vi "数据主动和反控发送.vi"() -> ()   [LabVIEW 2016, in "数据传输系统.lvlib"]
uses:
  <vilib>/ptbypt/NI_PtbyPt.lvlib
panel:
  out "QN":string
  out "队列中元素数量":i32
  out "元素":cluster{"命令编码CN":string, "QN":string}[](array[cluster])
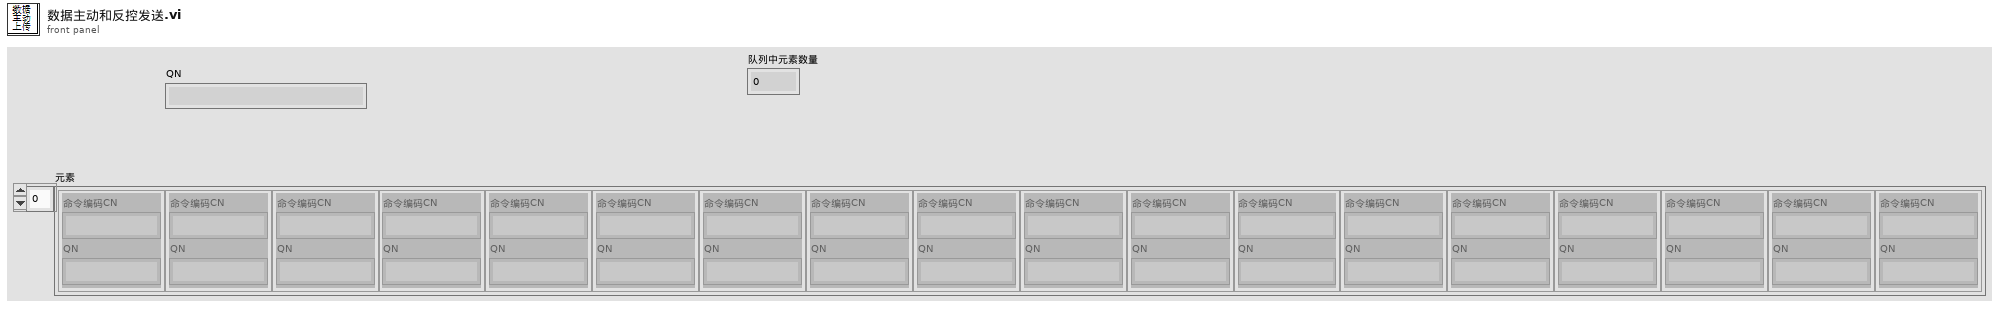
[diagram p1: front panel]
types:
  T1 = cluster{"setini":string, "sysini":string, "hechaini":string, "actualwrite":string, "actualread":string, "datasent":string, "反控命令信息队列":string, "反控与仪器交互":string}
  T2 = enum16{"00点", "01点", "02点", "03点", "04点", "05点", "06点", "07点", "08点", "09点", "10点", "11点", "12点", "13点", "14点", "15点", "16点", "17点", "18点", "19点", "20点", "21点", "22点", "23点"}
  T3 = enum16{"关闭", "星期日", "星期一", "星期二", "星期三", "星期四", "星期五", "星期六"}
  T4 = typedef "LVDateTimeRec.ctl" = cluster{"秒数的小数部分":dbl, "秒":i32, "分":i32, "时":i32, "日":i32, "月":i32, "年":i32, "天数（周）":i32, "天数（年）":i32, "DST":i32}
  T5 = cluster{"[0]":string, "[1]":string, "[2]":string, "[3]":string, "[4]":string, "[5]":string, "[6]":string, "[7]":string, "[8]":string, "[9]":string, "[10]":string, "[11]":string, "[12]":string, "[13]":string, "[14]":string, "[15]":string, "[16]":string, "[17]":string, "[18]":string, "[19]":string, "[20]":string, "[21]":string, "[22]":string, "[23]":string, "[24]":string, "[25]":string, "[26]":string, "[27]":string, "[28]":string, "[29]":string, "[30]":string}
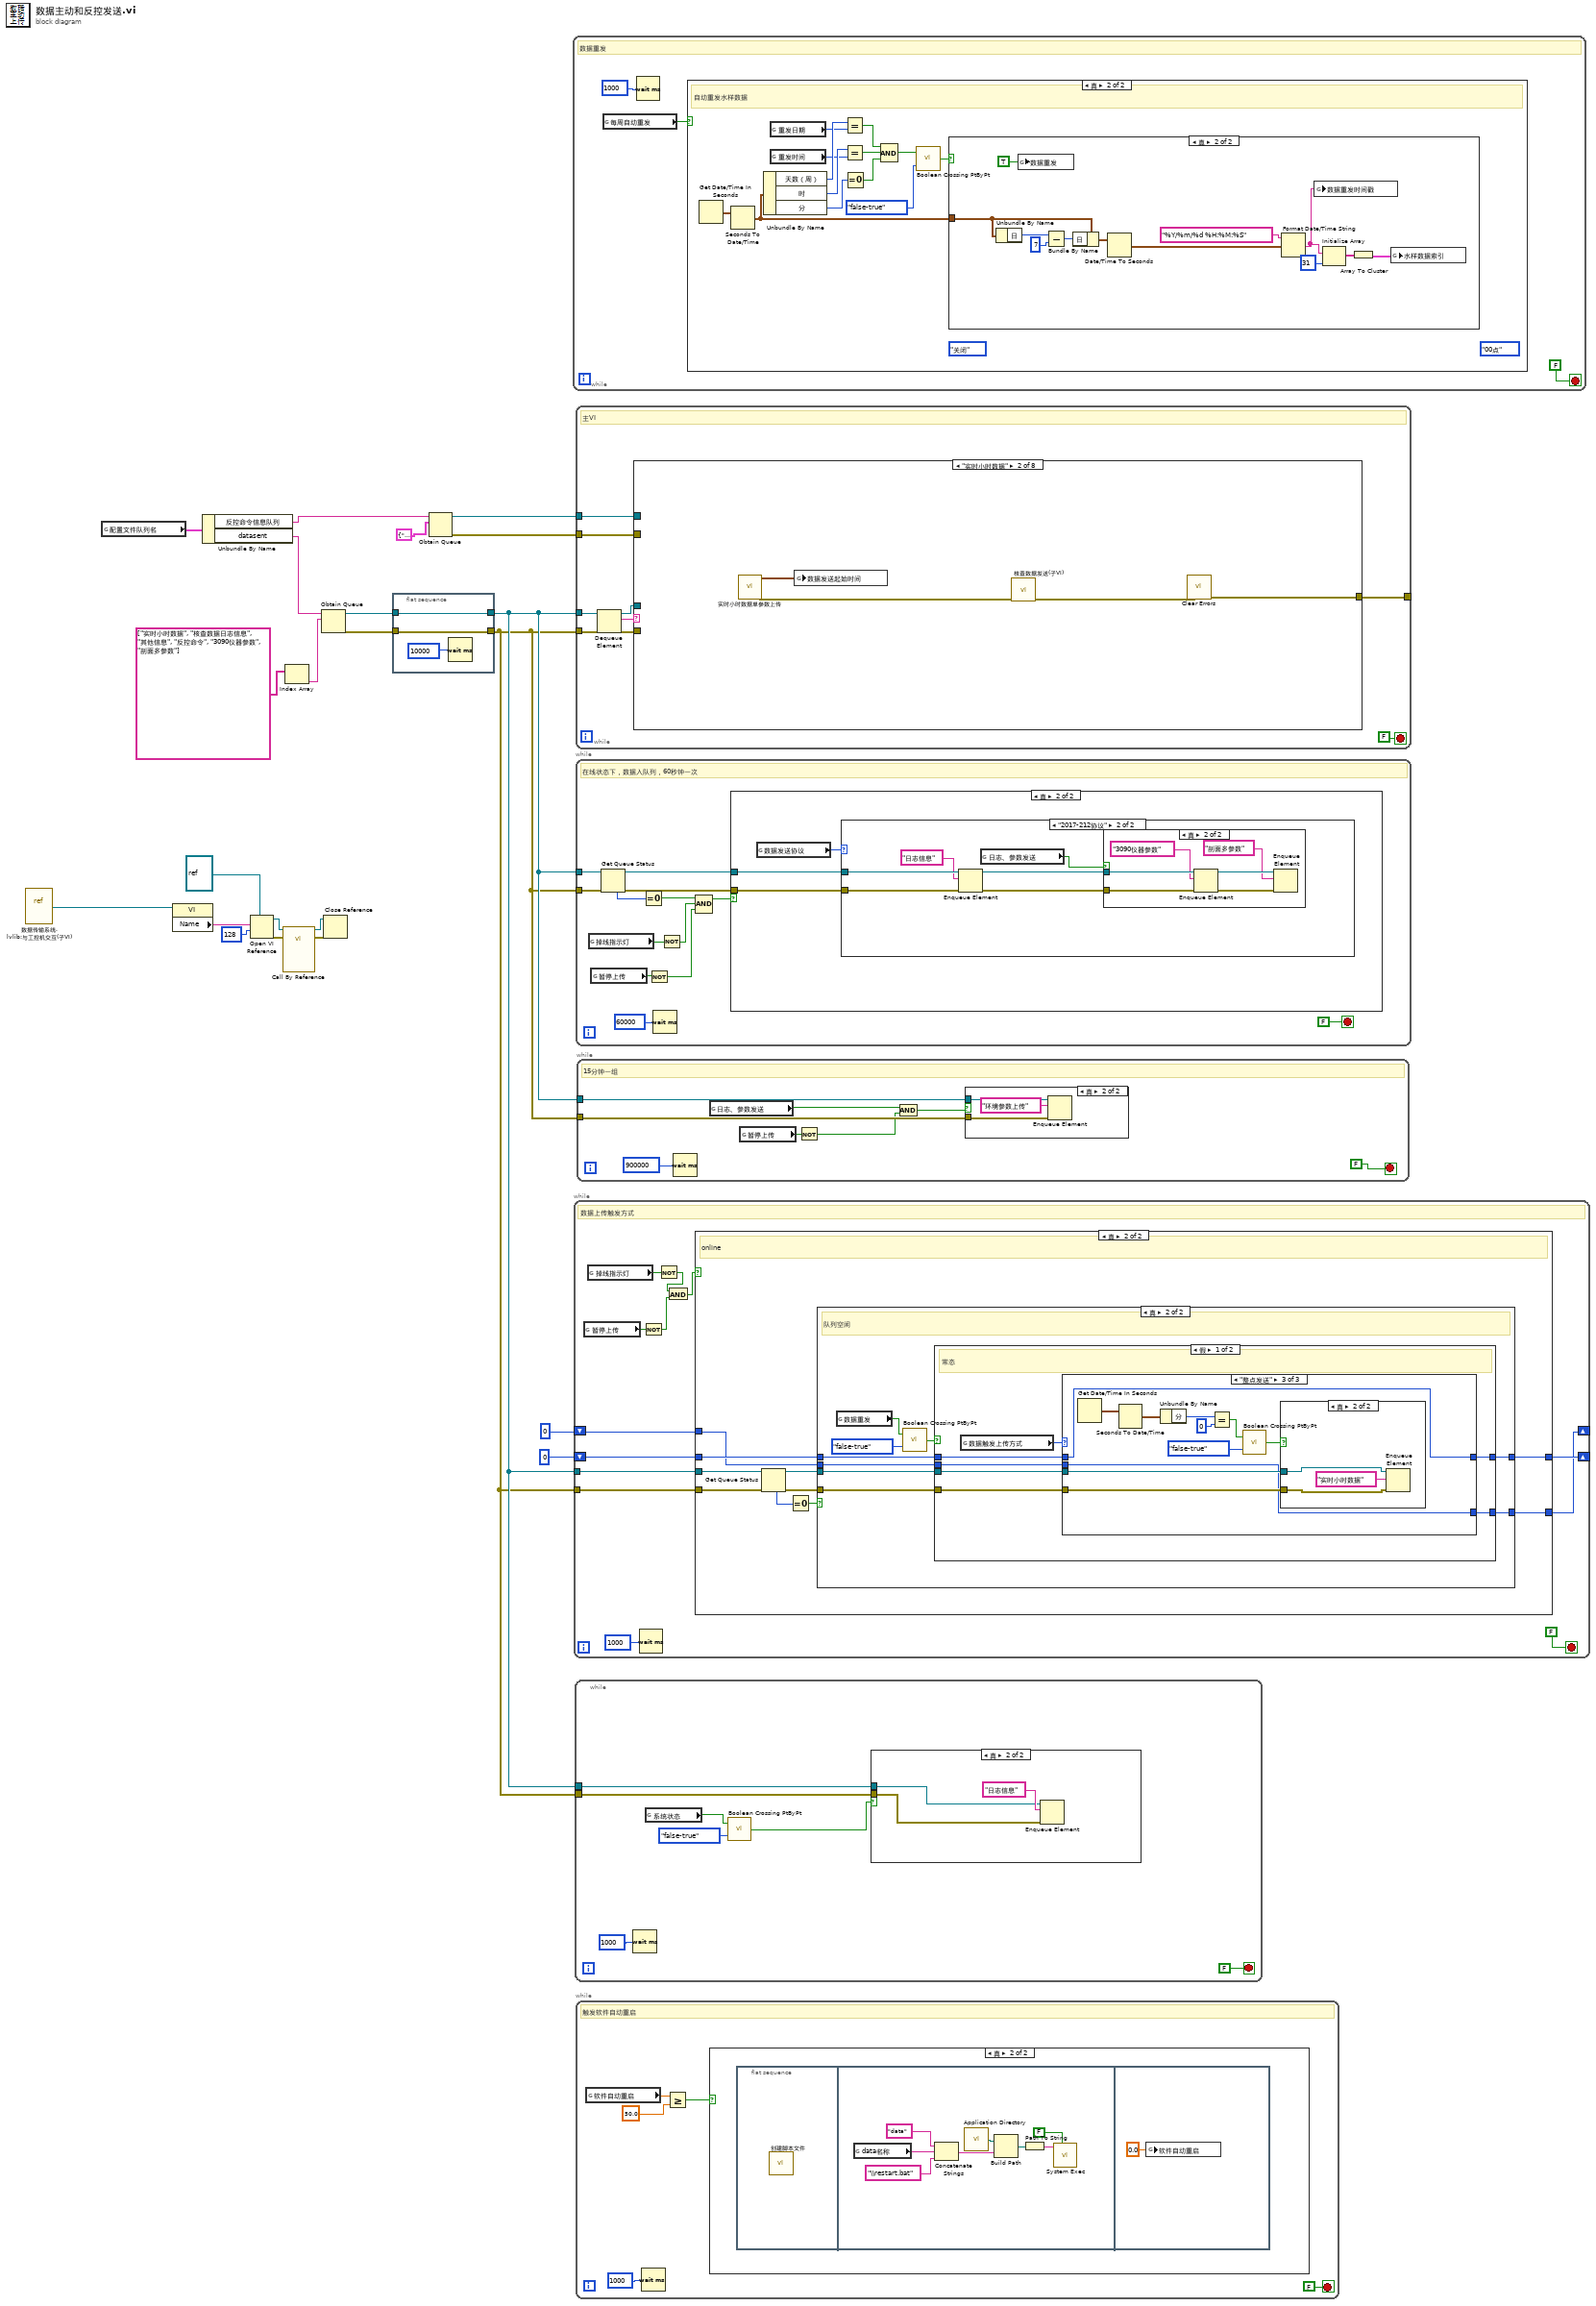
[diagram p0: block diagram]
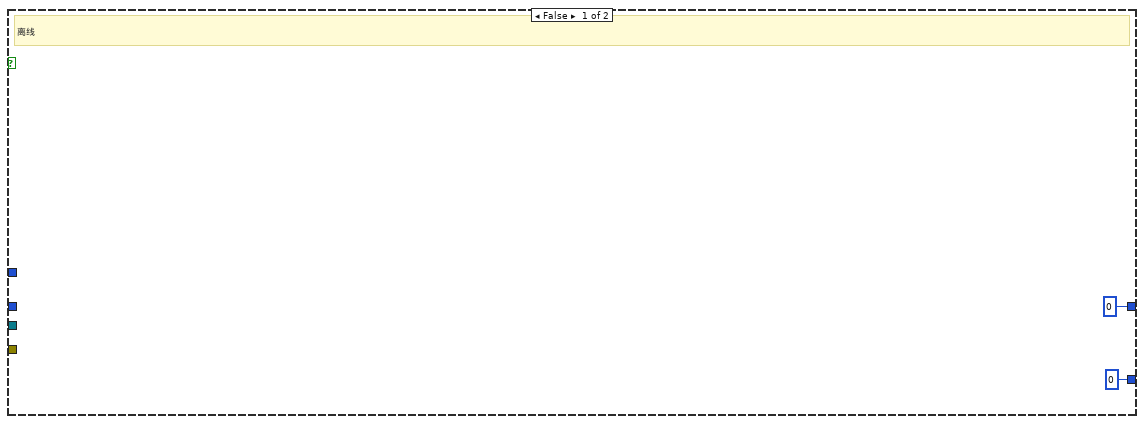
[diagram p4: hidden frame]
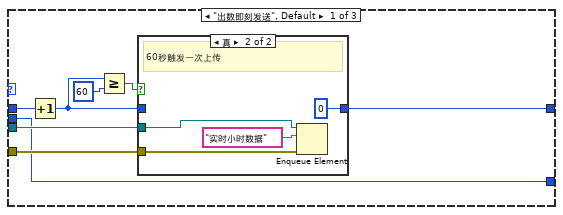
[diagram p6: hidden frame]
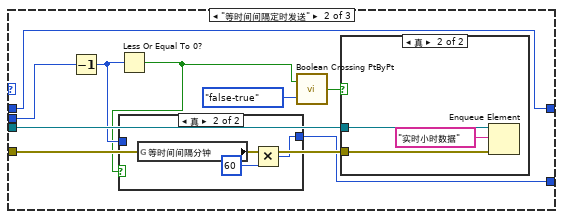
[diagram p8: hidden frame]
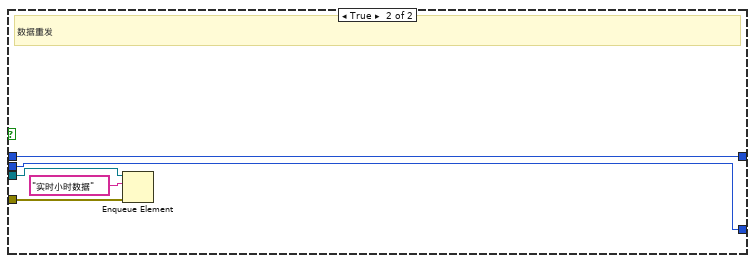
[diagram p12: hidden frame]
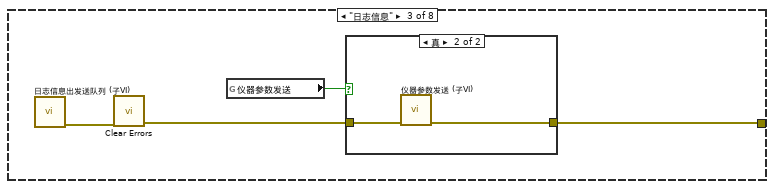
[diagram p20: hidden frame]
diagram:
  n1 = vi-ref "数据传输系统.lvlib:与工控机交互(子VI).vi"() -> (w15:refnum<vi>)
  n2 = global read "断电保存全局.vi" "配置文件队列名"() -> (w3:T1)
  n3 = property class="VI"(reference=w15) -> ("Name"=w14:string)  [unwired: 1 in, 2 out]
  n4 = Unbundle By Name(w3) -> ("反控命令信息队列"=w2:string, "datasent"=w1:string)
  n5 = Open VI Reference(type specifier VI Refnum (for type only)=refnum<vi> refnum, vi path=w14, options=128 ("选项")) -> (vi reference=w12:refnum<vi>, error out=w10:errorcluster)  [unwired: 3 in]
  n6 = call-by-ref "?"(reference=w12, error in=w10) -> (reference out=w8:refnum<vi>, error out=w9:errorcluster)  [unwired: 12 in]
  n7 = Index Array(array=string[] ["实时小时数据", "核查数据日志信息", "其他信息", "反控命令", "3090仪器参数", "剖面多参数"]) -> (element=w16:string)  [unwired: 1 in]
  n8 = Obtain Queue(name (unnamed)=w1, element data type=w16) -> (queue out=w22:refnum<queue>, error out=w21:errorcluster)  [unwired: 3 in, 1 out]
  n9 = Close Reference(reference=w8, error in (no error)=w9) -> ()  [unwired: 1 out]
  n10 = flat-sequence {
    tunnel: w22 -> [w24]
    tunnel: [w24] -> w5
    tunnel: w21 -> [w23]
    tunnel: [w23] -> w4
    frame #0 {
      n11 = Wait (ms)(milliseconds to wait=u32 10000 ("等待时间（毫秒）")) -> ()  [unwired: 1 out]
    }
  }
  n12 = Obtain Queue(name (unnamed)=w2, element data type=cluster{"命令编码CN":string, "QN":string} {"命令编码CN"="", "QN"=""}) -> (queue out=w19:refnum<queue>, error out=w18:errorcluster)  [unwired: 3 in, 1 out]
  n13 = while {
    stop <- FALSE stop-if-true
    # "数据重发"
    n14 = global read "断电保存全局.vi" "每周自动重发"() -> (w27:bool)
    n15 = Wait (ms)(milliseconds to wait=u32 1000 ("等待时间（毫秒）")) -> ()  [unwired: 1 out]
    n16 = case shown="真" w27 {
      frame False {
      }
      frame True {
        (unwired) T2."00点"
        (unwired) T3."关闭"
        # "自动重发水样数据"
        n17 = Get Date/Time In Seconds() -> (seconds since 1Jan1904=w41:timestamp)
        n18 = Seconds To Date/Time(time stamp (now)=w41) -> (date time rec=w35:T4)  [unwired: 1 in]
        n19 = Unbundle By Name(w35) -> ("天数（周）"=w40:i32, "时"=w31:i32, "分"=w39:i32)
        n20 = global read "断电保存全局.vi" "重发日期"() -> (w30:T3)
        n21 = global read "断电保存全局.vi" "重发时间"() -> (w29:T2)
        n22 = Equal?(x=w40, y=w30) -> (x = y?=w38:bool)
        n23 = Equal?(x=w31, y=w29) -> (x = y?=w37:bool)
        n24 = Equal To 0?(x=w39) -> (x = 0?=w36:bool)
        n25 = Compound Arithmetic op=AND ("复合运算")(w38, w37, w36) -> (w34:bool)
        n26 = call <vilib>:"Boolean Crossing PtByPt.vi"("direction"=enum16{"either", "false-true", "true-false"}."false-true", "input"=w34) -> ("crossing"=w33:bool)  [unwired: 1 in]
        n27 = case shown="真" w33 {
          tunnel: w35 -> [_ w49]
          frame False {
          }
          frame True {
            n28 = Unbundle By Name(w49) -> ("日"=w52:i32)
            n29 = global write "断电保存全局.vi" "数据重发"(TRUE ("数据重发")) -> ()
            n30 = Subtract(x=w52, y=7) -> (x-y=w50:i32)
            n31 = Bundle By Name(cluster=w49, "日"=w50) -> (w53:T4)
            n32 = Date/Time To Seconds(2:w53) -> (0:w48:timestamp)  [unwired: 1 in]
            n33 = Format Date/Time String(time format string (%c)="%Y/%m/%d %H:%M:%S" ("时间格式字符串(%c)"), seconds (now)=w48) -> (date/time string=w42:string)  [unwired: 1 in]
            n34 = global write "断电保存全局.vi" "数据重发时间戳"(w42) -> ()
            n35 = Initialize Array(w42, 31 ("维数大小")) -> (w44:string[])
            n36 = Array To Cluster(array=w44) -> (cluster=w43:T5)
            n37 = global write "全局 水样时间.vi" "水样数据索引"(w43) -> ()
          }
        }
      }
    }
  }
  n38 = while {
    tunnel: w5 -> [w61]
    tunnel: w4 -> [w60]
    shift-right: [w63] -> _
    shift-left: 0 -> [w64]
    shift-right: [w54] -> _
    shift-left: 0 -> [w55]
    stop <- FALSE stop-if-true
    # "数据上传触发方式"
    n39 = global read "断电保存全局.vi" "暂停上传"() -> (w58:bool)
    n40 = global read "全局 数据发送重叠.vi" "掉线指示灯"() -> (w65:bool)
    n41 = Wait (ms)(milliseconds to wait=u32 1000 ("等待时间（毫秒）")) -> ()  [unwired: 1 out]
    n42 = Not(x=w58) -> (.not. x?=w57:bool)
    n43 = Not(x=w65) -> (.not. x?=w59:bool)
    n44 = And(x=w59, y=w57) -> (x .and. y?=w56:bool)
    n45 = case shown="真" w56 {
      tunnel: w64 -> [_ w78]
      tunnel: [0 w77] -> w63
      tunnel: w61 -> [_ w75]
      tunnel: w60 -> [_ w74]
      tunnel: w55 -> [_ w70]
      tunnel: [0 w69] -> w54
      frame False {
        # "离线"
      }
      frame True {
        # "online"
        n46 = Get Queue Status(queue=w75, error in (no error)=w74) -> (queue out=w72:refnum<queue>, error out=w71:errorcluster, # elements in queue=w76:i32)  [unwired: 1 in, 5 out]
        n47 = Equal To 0?(x=w76) -> (x = 0?=w73:bool)
        n48 = case shown="真" w73 {
          tunnel: w72 -> [_ w89]
          tunnel: w71 -> [_ w88]
          tunnel: w78 -> [w80 w87]
          tunnel: [w80 w86] -> w77
          tunnel: w70 -> [w79 w82]
          tunnel: [w79 w81] -> w69
          frame False {
            # "队列忙碌中"
          }
          frame True {
            # "队列空闲"
            n49 = global read "断电保存全局.vi" "数据重发"() -> (w84:bool)
            n50 = call <vilib>:"Boolean Crossing PtByPt.vi"("direction"=enum16{"either", "false-true", "true-false"}."false-true", "input"=w84) -> ("crossing"=w83:bool)  [unwired: 1 in]
            n51 = case shown="假" w83 {
              tunnel: w89 -> [w96 w143]
              tunnel: w88 -> [w95 w142]
              tunnel: w87 -> [w93 w141]
              tunnel: [w92 w141] -> w86
              tunnel: w82 -> [w91 w140]
              tunnel: [w90 w140] -> w81
              frame False {
                # "常态"
                n52 = global read "断电保存全局.vi" "数据触发上传方式"() -> (w94:enum16{"出数即刻发送", "等时间间隔定时发送", "整点发送"})
                n53 = case shown="\"整点发送\"" w94 {
                  tunnel: w96 -> [w99 w117 w130]
                  tunnel: w95 -> [w98 w116 w129]
                  tunnel: w93 -> [w104 w118 w128]
                  tunnel: [w100 w118 w128] -> w92
                  tunnel: w91 -> [w97 w113 w126]
                  tunnel: [w97 w112 w126] -> w90
                  frame "出数即刻发送", Default {
                    n54 = Increment(x=w104) -> (x+1=w101:i32)
                    n55 = Greater Or Equal?(x=w101, y=60) -> (x >= y?=w102:bool)
                    n56 = case shown="真" w102 {
                      tunnel: w101 -> [w105 _]
                      tunnel: [w105 0] -> w100
                      tunnel: w99 -> [_ w107]
                      tunnel: w98 -> [_ w106]
                      frame False {
                      }
                      frame True {
                        # "60秒触发一次上传"
                        n57 = Enqueue Element(queue=w107, element="实时小时数据" ("元素"), error in (no error)=w106) -> ()  [unwired: 1 in, 3 out]
                      }
                    }
                  }
                  frame "等时间间隔定时发送" {
                    n58 = Decrement(x=w113) -> (x-1=w111:i32)
                    n59 = Less Or Equal To 0?(x=w111) -> (x <= 0?=w110:bool)
                    n60 = case shown="真" w110 {
                      tunnel: w111 -> [w119 _]
                      tunnel: [w119 w120] -> w112
                      frame False {
                      }
                      frame True {
                        n61 = global read "断电保存全局.vi" "等时间间隔分钟"() -> (w121:i32)
                        n62 = Multiply(x=w121, y=60) -> (x*y=w120:i32)
                      }
                    }
                    n63 = call <vilib>:"Boolean Crossing PtByPt.vi"("direction"=enum16{"either", "false-true", "true-false"}."false-true", "input"=w110) -> ("crossing"=w114:bool)  [unwired: 1 in]
                    n64 = case shown="真" w114 {
                      tunnel: w117 -> [_ w124]
                      tunnel: w116 -> [_ w123]
                      frame False {
                      }
                      frame True {
                        n65 = Enqueue Element(queue=w124, element="实时小时数据" ("元素"), error in (no error)=w123) -> ()  [unwired: 1 in, 3 out]
                      }
                    }
                  }
                  frame "整点发送" {
                    n66 = Get Date/Time In Seconds() -> (seconds since 1Jan1904=w135:timestamp)
                    n67 = Seconds To Date/Time(time stamp (now)=w135) -> (date time rec=w136:T4)  [unwired: 1 in]
                    n68 = Unbundle By Name(w136) -> ("分"=w134:i32)
                    n69 = Equal?(x=w134, y=0) -> (x = y?=w132:bool)
                    n70 = call <vilib>:"Boolean Crossing PtByPt.vi"("direction"=enum16{"either", "false-true", "true-false"}."false-true", "input"=w132) -> ("crossing"=w127:bool)  [unwired: 1 in]
                    n71 = case shown="真" w127 {
                      tunnel: w130 -> [_ w138]
                      tunnel: w129 -> [_ w137]
                      frame False {
                      }
                      frame True {
                        n72 = Enqueue Element(queue=w138, element="实时小时数据" ("元素"), error in (no error)=w137) -> ()  [unwired: 1 in, 3 out]
                      }
                    }
                  }
                }
              }
              frame True {
                # "数据重发"
                n73 = Enqueue Element(queue=w143, element="实时小时数据" ("元素"), error in (no error)=w142) -> ()  [unwired: 1 in, 3 out]
              }
            }
          }
        }
      }
    }
  }
  n74 = while {
    tunnel: w5 -> [w146]
    tunnel: w4 -> [w145]
    stop <- FALSE stop-if-true
    n75 = Wait (ms)(milliseconds to wait=u32 1000 ("等待时间（毫秒）")) -> ()  [unwired: 1 out]
    n76 = global read "全局1.vi" "系统状态"() -> (w149:bool)
    n77 = call <vilib>:"Boolean Crossing PtByPt.vi"("direction"=enum16{"either", "false-true", "true-false"}."false-true", "input"=w149) -> ("crossing"=w147:bool)  [unwired: 1 in]
    n78 = case shown="真" w147 {
      tunnel: w146 -> [_ w153]
      tunnel: w145 -> [_ w152]
      frame False {
      }
      frame True {
        n79 = Enqueue Element(queue=w153, element="日志信息" ("元素"), error in (no error)=w152) -> ()  [unwired: 1 in, 3 out]
      }
    }
  }
  n80 = while {
    tunnel: w5 -> [w157]
    tunnel: w4 -> [w156]
    tunnel: w19 -> [w159]
    tunnel: w18 -> [w158]
    tunnel: [w155] -> _
    stop <- FALSE stop-if-true
    # "主VI"
    n81 = Dequeue Element(queue=w157, error in (no error)=w156) -> (queue out=w161:refnum<queue>, element=w162:string, error out=w160:errorcluster)  [unwired: 1 in, 1 out]
    n82 = case shown="\"实时小时数据\"" w162 {
      tunnel: w161 -> [_ _ _ _ w176 _ _ _]
      tunnel: w160 -> [_ _ _ _ w175 _ _ _]
      tunnel: w159 -> [_ _ _ _ w186 _ _ _]
      tunnel: w158 -> [_ _ _ _ w185 _ _ _]
      tunnel: [_ w166 w169 _ _ w195 w198 w200] -> w155
      frame Default {
      }
      frame "实时小时数据" {
        n83 = call "实时小时数据单参数上传.vi"() -> ("数据发送起始时间"=w167:timestamp, "error out"=w165:errorcluster)  [unwired: 14 in]
        n84 = global write "全局1.vi" "数据发送起始时间"(w167) -> ()
        n85 = call "核查数据发送(子VI).vi"("错误输入"=w165) -> ("错误输出"=w164:errorcluster)  [unwired: 10 in]
        n86 = call <vilib>:"Clear Errors.vi"("error in (no error)"=w164) -> ("error out"=w166:errorcluster)  [unwired: 5 in, 1 out]
      }
      frame "日志信息" {
        n87 = call "日志信息出发送队列 (子VI).vi"() -> ("错误输出"=w171:errorcluster)  [unwired: 11 in]
        n88 = call <vilib>:"Clear Errors.vi"("error in (no error)"=w171) -> ("error out"=w170:errorcluster)  [unwired: 5 in, 1 out]
        n89 = global read "断电保存全局.vi" "仪器参数发送"() -> (w168:bool)
        n90 = case shown="真" w168 {
          tunnel: w170 -> [w172 w174]
          tunnel: [w172 w173] -> w169
          frame False {
          }
          frame True {
            n91 = call "仪器参数发送 (子VI).vi"("错误输入"=w174) -> ("错误输出"=w173:errorcluster)  [unwired: 10 in]
          }
        }
      }
      frame "其他信息" {
      }
      frame "反控命令" {
        n92 = Get Queue Status(queue=w186, return elements? (F)=TRUE ("返回元素？(F)"), error in (no error)=w185) -> (# elements in queue=→"队列中元素数量":i32, elements=→"元素":cluster{"命令编码CN":string, "QN":string}[])  [unwired: 6 out]
        n93 = Dequeue Element(queue=w186, error in (no error)=w185) -> (element=w182:cluster{"命令编码CN":string, "QN":string})  [unwired: 1 in, 3 out]
        n94 = Unbundle By Name(w182) -> ("命令编码CN"=w181:string, "QN"=w180:string)
        "QN" <- w180
        n95 = global read "全局1.vi" "数据"() -> (w184:string)
        n96 = call "读取反控数据解析(子VI).vi"("数据"=w184, "命令编码CN"=w181) -> ("反控命令错误？"=w183:bool)  [unwired: 8 in, 1 out]
        n97 = case shown="假" w183 {
          tunnel: w180 -> [w190 _]
          tunnel: w176 -> [w188 _]
          tunnel: w175 -> [w187 _]
          frame False {
            # "反控命令正确"
            n98 = call "反控数据上传(子VI).vi"("QN"=w190) -> ("error out"=w189:errorcluster)  [unwired: 10 in]
            n99 = case shown="无错误" w189 {
              tunnel: w188 -> [w193 _]
              tunnel: w187 -> [w192 _]
              frame No Error {
                n100 = Enqueue Element(queue=w193, element="核查数据日志信息" ("元素"), error in (no error)=w192) -> ()  [unwired: 1 in, 3 out]
              }
              frame Error {
              }
            }
          }
          frame True {
            # "反控命令错误"
          }
        }
      }
      frame "3090仪器参数" {
        n101 = global read "断电保存全局.vi" "应用环境"() -> (w194:enum16{"STD", "GB212"})
        n102 = case shown="\"STD\", 默认" w194 {
          tunnel: [w196 _] -> w195
          frame "STD", Default {
            n103 = call "3090仪器参数上传.vi"() -> ("error out"=w196:errorcluster)  [unwired: 15 in]
          }
          frame "GB212" {
          }
        }
      }
      frame "剖面多参数" {
        n104 = global read "断电保存全局.vi" "应用环境"() -> (w197:enum16{"STD", "GB212"})
        n105 = case shown="\"STD\", 默认" w197 {
          tunnel: [w199 _] -> w198
          frame "STD", Default {
            n106 = call "剖面多参数上传.vi"() -> ("error out"=w199:errorcluster)  [unwired: 15 in]
          }
          frame "GB212" {
          }
        }
      }
      frame "环境参数上传" {
        n107 = call "环境参数上传.vi"() -> ("error out"=w200:errorcluster)  [unwired: 15 in]
      }
    }
  }
  n108 = while {
    tunnel: w5 -> [w213]
    tunnel: w4 -> [w212]
    stop <- FALSE stop-if-true
    # "在线状态下，数据入队列，60秒钟一次"
    n109 = global read "全局 数据发送重叠.vi" "掉线指示灯"() -> (w206:bool)
    n110 = global read "断电保存全局.vi" "暂停上传"() -> (w202:bool)
    n111 = Get Queue Status(queue=w213, error in (no error)=w212) -> (queue out=w210:refnum<queue>, error out=w209:errorcluster, # elements in queue=w211:i32)  [unwired: 1 in, 5 out]
    n112 = Equal To 0?(x=w211) -> (x = 0?=w204:bool)
    n113 = Not(x=w202) -> (.not. x?=w201:bool)
    n114 = Wait (ms)(milliseconds to wait=u32 60000 ("等待时间（毫秒）")) -> ()  [unwired: 1 out]
    n115 = Not(x=w206) -> (.not. x?=w203:bool)
    n116 = Compound Arithmetic op=AND ("复合运算")(w204, w203, w201) -> (w205:bool)
    n117 = case shown="真" w205 {
      tunnel: w210 -> [_ w216]
      tunnel: w209 -> [_ w215]
      frame False {
      }
      frame True {
        n118 = global read "断电保存全局.vi" "数据发送协议"() -> (w214:enum16{"2005-212协议", "2017-212协议"})
        n119 = case shown="\"2017-212协议\"" w214 {
          tunnel: w216 -> [_ w222]
          tunnel: w215 -> [_ w221]
          frame "2005-212协议", Default {
          }
          frame "2017-212协议" {
            n120 = Enqueue Element(queue=w222, element="日志信息" ("元素"), error in (no error)=w221) -> (queue out=w219:refnum<queue>, error out=w218:errorcluster)  [unwired: 1 in, 1 out]
            n121 = global read "断电保存全局.vi" "日志、参数发送"() -> (w217:bool)
            n122 = case shown="真" w217 {
              tunnel: w219 -> [_ w228]
              tunnel: w218 -> [_ w227]
              frame False {
              }
              frame True {
                n123 = Enqueue Element(queue=w228, element="3090仪器参数" ("元素"), error in (no error)=w227) -> (queue out=w225:refnum<queue>, error out=w224:errorcluster)  [unwired: 1 in, 1 out]
                n124 = Enqueue Element(queue=w225, element="剖面多参数" ("元素"), error in (no error)=w224) -> ()  [unwired: 1 in, 3 out]
              }
            }
          }
        }
      }
    }
  }
  n125 = while {
    stop <- FALSE stop-if-true
    # "触发软件自动重启"
    n126 = global read "全局1.vi" "软件自动重启"() -> (w231:dbl)
    n127 = Wait (ms)(milliseconds to wait=u32 1000 ("等待时间（毫秒）")) -> ()  [unwired: 1 out]
    n128 = Greater Or Equal?(x=w231, y=50.0) -> (x >= y?=w229:bool)
    n129 = case shown="真" w229 {
      frame False {
      }
      frame True {
        n130 = flat-sequence {
          frame #0 {
            n131 = call "创建脚本文件.vi"() -> ()  [unwired: 11 in, 1 out]
          }
          frame #1 {
            n132 = global read "断电保存全局.vi" "data名称"() -> (w236:string)
            n133 = Concatenate Strings("data" ("名称或相对路径"), w236, "\\restart.bat" ("字符串")) -> (w234:string)
            n134 = call <vilib>:"Application Directory.vi"() -> ("Application Directory"=w240:path)
            n135 = Build Path(base path=w240, name or relative path=w234) -> (appended path=w241:path)
            n136 = Path To String(path=w241) -> (string=w238:string)
            n137 = call <vilib>:"System Exec.vi"("wait until completion? (T)"=FALSE, "command line"=w238) -> ()  [unwired: 6 in, 4 out]
          }
          frame #2 {
            n138 = global write "全局1.vi" "软件自动重启"(0.0 ("软件自动重启")) -> ()
          }
        }
      }
    }
  }
  n139 = while {
    tunnel: w5 -> [w248]
    tunnel: w4 -> [w247]
    stop <- FALSE stop-if-true
    # "15分钟一组"
    n140 = Wait (ms)(milliseconds to wait=u32 900000 ("等待时间（毫秒）")) -> ()  [unwired: 1 out]
    n141 = global read "断电保存全局.vi" "日志、参数发送"() -> (w245:bool)
    n142 = global read "断电保存全局.vi" "暂停上传"() -> (w246:bool)
    n143 = Not(x=w246) -> (.not. x?=w244:bool)
    n144 = And(x=w245, y=w244) -> (x .and. y?=w243:bool)
    n145 = case shown="真" w243 {
      tunnel: w248 -> [_ w252]
      tunnel: w247 -> [_ w251]
      frame False {
      }
      frame True {
        n146 = Enqueue Element(queue=w252, element="环境参数上传" ("元素"), error in (no error)=w251) -> ()  [unwired: 1 in, 3 out]
      }
    }
  }
